vi "Ammeter Zero (648X).vi"(8 "error in (no error)":errorcluster, 11 "VISA resource name in":refnum<visa-resource-name>) -> (0 "error out":errorcluster, 3 "VISA resource name out":refnum<visa-resource-name>)   [LabVIEW 2016, in "Hall Effect Library.lvlib"]
uses:
  Hall Effect Library.lvlib
  <instrlib>/Keithley 648X/Keithley 648X.lvlib
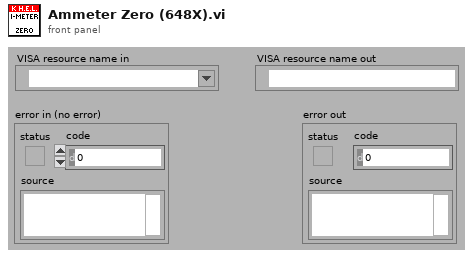
[diagram p1: front panel]
types:
  T1 = enum16{"Auto", "2 nA", "20 nA", "200 nA", "2 uA", "20 uA", "200 uA", "2 mA", "20 mA"}
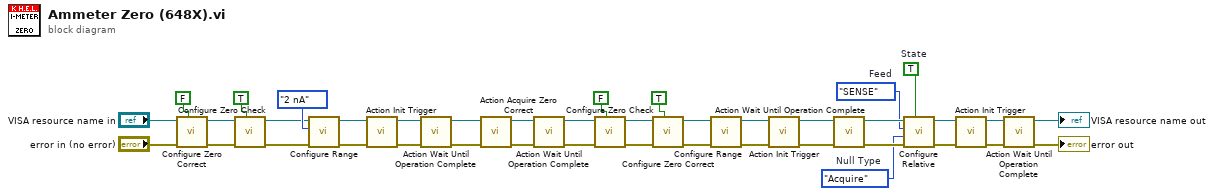
[diagram p0: block diagram]
diagram:
  w7 = TRUE  # State
  w9 = enum16{"Acquire", "Offset"}."Acquire"  # Null Type
  w8 = enum16{"SENSE", "CALC"}."SENSE"  # Feed
  n1 = call <instrlib>:"Configure Zero Correct.vi"("Zero Correct (T: On)"=FALSE, "error in (no error)"="error in (no error)", "VISA resource name"="VISA resource name in") -> ("error out"=w39:errorcluster, "VISA resource name out"=w40:refnum<visa-resource-name>)  [unwired: 7 out]
  n2 = call <instrlib>:"Configure Zero Check.vi"("Zero Check (T: On)"=TRUE, "error in (no error)"=w39, "VISA resource name"=w40) -> ("error out"=w27:errorcluster, "VISA resource name out"=w26:refnum<visa-resource-name>)  [unwired: 7 out]
  n3 = call <instrlib>:"Configure Range.vi"("error in"=w27, "Range (Auto)"=T1."2 nA", "VISA resource name"=w26) -> ("error out"=w29:errorcluster, "VISA resource name out"=w28:refnum<visa-resource-name>)  [unwired: 2 in, 5 out]
  n4 = call <instrlib>:"Action Init Trigger.vi"("error in (no error)"=w29, "VISA resource name"=w28) -> ("error out"=w20:errorcluster, "VISA resource name out"=w21:refnum<visa-resource-name>)  [unwired: 8 out]
  n5 = call <instrlib>:"Action Wait Until Operation Complete.vi"("error in"=w20, "VISA resource name"=w21) -> ("error out"=w18:errorcluster, "VISA resource name out"=w19:refnum<visa-resource-name>)  [unwired: 1 in, 7 out]
  n6 = call <instrlib>:"Action Acquire Zero Correct.vi"("error in (no error)"=w18, "VISA resource name"=w19) -> ("error out"=w17:errorcluster, "VISA resource name out"=w16:refnum<visa-resource-name>)  [unwired: 8 out]
  n7 = call <instrlib>:"Action Wait Until Operation Complete.vi"("error in"=w17, "VISA resource name"=w16) -> ("error out"=w12:errorcluster, "VISA resource name out"=w13:refnum<visa-resource-name>)  [unwired: 1 in, 7 out]
  n8 = call <instrlib>:"Configure Zero Check.vi"("Zero Check (T: On)"=FALSE, "error in (no error)"=w12, "VISA resource name"=w13) -> ("error out"=w30:errorcluster, "VISA resource name out"=w31:refnum<visa-resource-name>)  [unwired: 7 out]
  n9 = call <instrlib>:"Configure Zero Correct.vi"("Zero Correct (T: On)"=TRUE, "error in (no error)"=w30, "VISA resource name"=w31) -> ("error out"=w36:errorcluster, "VISA resource name out"=w37:refnum<visa-resource-name>)  [unwired: 7 out]
  n10 = call <instrlib>:"Configure Range.vi"("error in"=w36, "VISA resource name"=w37) -> ("error out"=w23:errorcluster, "VISA resource name out"=w22:refnum<visa-resource-name>)  [unwired: 3 in, 5 out]
  n11 = call <instrlib>:"Action Init Trigger.vi"("error in (no error)"=w23, "VISA resource name"=w22) -> ("error out"=w15:errorcluster, "VISA resource name out"=w14:refnum<visa-resource-name>)  [unwired: 8 out]
  n12 = call <instrlib>:"Action Wait Until Operation Complete.vi"("error in"=w15, "VISA resource name"=w14) -> ("error out"=w11:errorcluster, "VISA resource name out"=w10:refnum<visa-resource-name>)  [unwired: 1 in, 7 out]
  n13 = call <instrlib>:"Configure Relative.vi"("State"=w7, "error in"=w11, "Null Type"=w9, "Feed"=w8, "VISA resource name"=w10) -> ("error out"=w6:errorcluster, "VISA resource name out"=w5:refnum<visa-resource-name>)  [unwired: 2 in, 3 out]
  n14 = call <instrlib>:"Action Init Trigger.vi"("error in (no error)"=w6, "VISA resource name"=w5) -> ("error out"=w4:errorcluster, "VISA resource name out"=w3:refnum<visa-resource-name>)  [unwired: 8 out]
  n15 = call <instrlib>:"Action Wait Until Operation Complete.vi"("error in"=w4, "VISA resource name"=w3) -> ("error out"=→"error out":errorcluster, "VISA resource name out"=→"VISA resource name out":refnum<visa-resource-name>)  [unwired: 1 in, 7 out]
